vi "脉冲生成_基于时钟滴答_有限.vi"() -> ()   [LabVIEW 2013]
uses:
  <userlib>/ArtDAQ/_SubVI/ArtDAQ_CreateCOPulseChanTicks.vi
  <userlib>/ArtDAQ/_SubVI/ArtDAQ_CfgImplicitTiming.vi
  <userlib>/ArtDAQ/_SubVI/ArtDAQ_CfgDigEdgeStartTrig.vi
panel:
  in  "时钟滴答源":string="/Dev1/PFI1"
  in  "TriggerMode":enum32{"No Trigger", "DigStartTrig"}(tab)
  in  "触发边沿":i32(ring)=10280 items=["上升"=10280, "下降"=10171]
  in  "触发源":string(combo)="/Dev1/PFI2"
  in  "每通道采样":i32=1000
  in  "Stop":bool
  in  "计数器":string="Dev1/ctr0"
  in  "高滴答数":i32=100
  in  "低滴答数":i32=100
  out "错误输出":errorcluster
  # "通道属性"
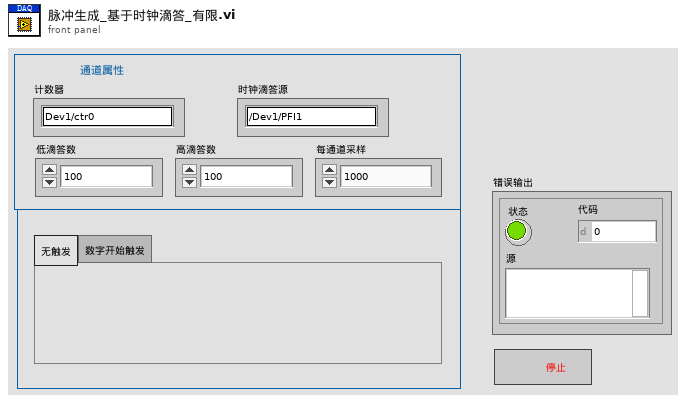
[diagram p1: front panel]
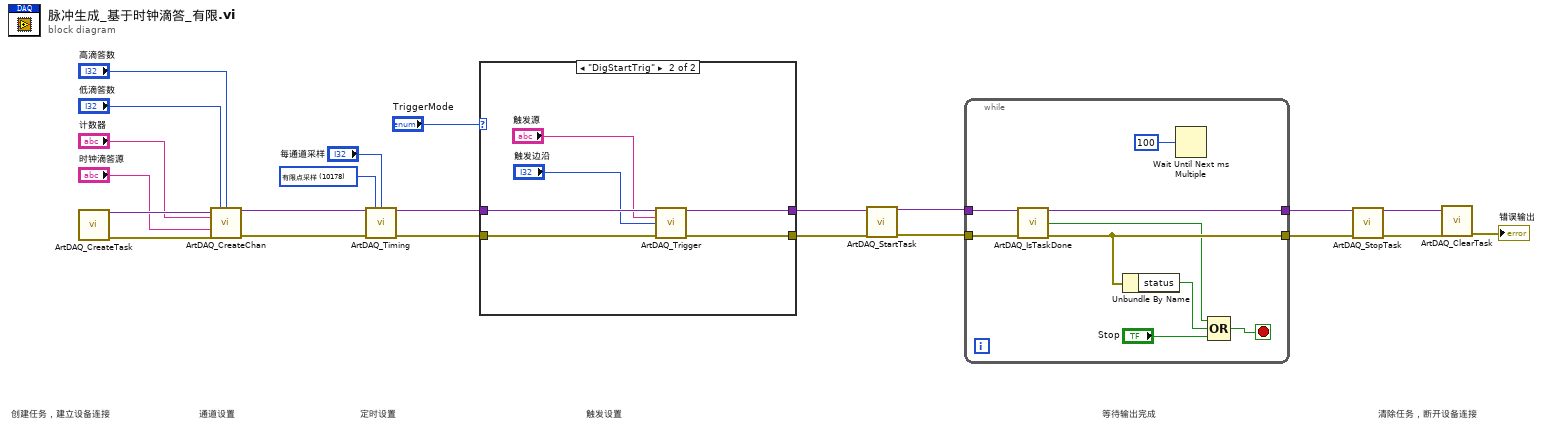
[diagram p0: block diagram]
diagram:
  w11 = 10178 items=["有限点采样"=10178, "连续采样"=10123] ("SampleMode")
  # "清除任务，断开设备连接"
  # "等待输出完成"
  # "定时设置"
  # "触发设置"
  # "通道设置"
  # "创建任务，建立设备连接"
  n1 = call <userlib>:"ArtDAQ_CreateTask.vi"() -> ("任务句柄"=w22:variant, "错误输出"=w21:errorcluster)  [unwired: 14 in]
  n2 = call-poly <userlib>:"ArtDAQ_CreateChan.vi"("任务句柄"=w22, "低时钟滴答"="低滴答数", "高时钟滴答"="高滴答数", "计数器"="计数器", "时钟滴答源"="时钟滴答源", "错误输入"=w21) -> ("任务句柄"=w13:variant, "错误输出"=w12:errorcluster)  [unwired: 8 in]
  n3 = call-poly <userlib>:"ArtDAQ_Timing.vi"("任务句柄"=w13, "采样模式"=w11, "每通道采样数"="每通道采样", "错误输入"=w12) -> ("任务句柄"=w8:variant, "错误输出"=w7:errorcluster)  [unwired: 10 in]
  n4 = case shown="\"DigStartTrig\"" "TriggerMode" {
    tunnel: w8 -> [w24 w30]
    tunnel: [w24 w29] -> w6
    tunnel: [w23 w28] -> w4
    tunnel: w7 -> [w23 w27]
    frame "No Trigger", Default {
    }
    frame "DigStartTrig" {
      n5 = call-poly <userlib>:"ArtDAQ_Trigger.vi"("任务句柄"=w30, "触发源"="触发源", "边沿"="触发边沿", "错误输入"=w27) -> ("任务句柄"=w29:variant, "错误输出"=w28:errorcluster)  [unwired: 10 in]
    }
  }
  n6 = call <userlib>:"ArtDAQ_StartTask.vi"("任务句柄"=w6, "错误输入"=w4) -> ("任务句柄"=w5:variant, "错误输出"=w3:errorcluster)  [unwired: 12 in]
  n7 = while {
    tunnel: [w39] -> w20
    tunnel: [w38] -> w18
    tunnel: w5 -> [w35]
    tunnel: w3 -> [w34]
    stop <- w33 stop-if-true
    n8 = call <userlib>:"ArtDAQ_IsTaskDone.vi"("任务句柄"=w35, "错误输入"=w34) -> ("任务句柄"=w39:variant, "完成任务？"=w31:bool, "错误输出"=w38:errorcluster)  [unwired: 11 in]
    n9 = Unbundle By Name(w38) -> ("status"=w37:bool)
    n10 = Wait Until Next ms Multiple(millisecond multiple=u32 100 ("毫秒倍数")) -> ()  [unwired: 1 out]
    n11 = Compound Arithmetic op=OR(w31, w37, "Stop") -> (w33:bool)
  }
  n12 = call <userlib>:"ArtDAQ_StopTask.vi"("任务句柄"=w20, "错误输入"=w18) -> ("任务句柄"=w19:variant, "错误输出"=w17:errorcluster)  [unwired: 12 in]
  n13 = call <userlib>:"ArtDAQ_ClearTask.vi"("任务句柄"=w19, "错误输入"=w17) -> ("错误输出"=→"错误输出":errorcluster)  [unwired: 13 in]
